vi "triangle_wave_2.vi"() -> ()   [LabVIEW 2017]
panel:
  out "x-y*floor(x/y)":dbl
  out "Waveform Chart":dbl(graph)
  in  "hz":i32
  in  "stop":bool
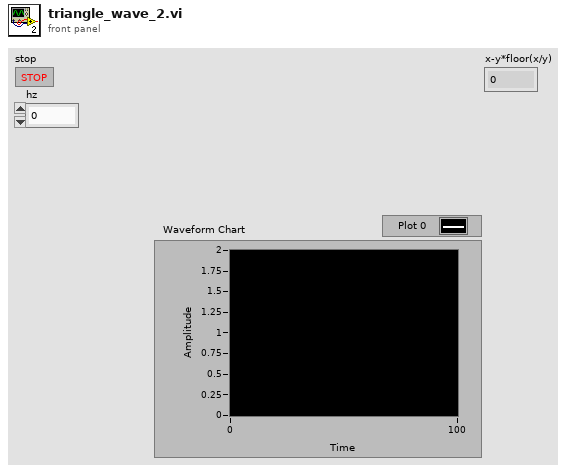
[diagram p1: front panel]
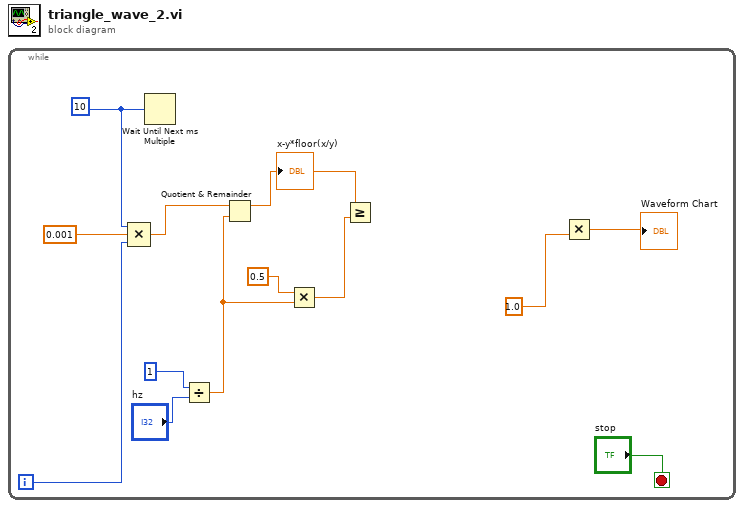
[diagram p0: block diagram]
diagram:
  n1 = while {
    i -> [w10]
    stop <- "stop" stop-if-true
    w12 = 10
    n2 = Compound Arithmetic op=MULTIPLY(w12, 0.001, w10) -> (w7:dbl)
    n3 = Wait Until Next ms Multiple(millisecond multiple=w12) -> ()  [unwired: 1 out]
    n4 = Divide(x=1, y="hz") -> (x/y=w1:dbl)
    n5 = Quotient & Remainder(x=w7, y=w1) -> (x-y*floor(x/y)=w2:dbl)  [unwired: 1 out]
    "x-y*floor(x/y)" <- w2
    n6 = Multiply(x=0.5, y=w1) -> (x*y=w5:dbl)
    n7 = Greater Or Equal?(x=w2, y=w5) -> ()  [unwired: 1 out]
    n8 = Multiply(y=1.0) -> (x*y=→"Waveform Chart":dbl)  [unwired: 1 in]
  }
